vi "Read SPD (pps).vi"(8 "error in (no error)":errorcluster, 11 "Motor in":refnum<class "Motor.lvclass">) -> (0 "error out":errorcluster, 1 "min speed in pps":dbl, 2 "max speed in pps":dbl, 3 "Motor out":refnum<class "Motor.lvclass">)   [LabVIEW 2016, in "Hardware.lvlib" / "Motor.lvlib" / "Motor.lvclass"]
uses:
  <userlib>/Common Components/Hardware/Motor/Motor/Motor.lvclass
  <userlib>/Common Components/Hardware/Motor/Motor/Motor.lvclass/Motor.ctl
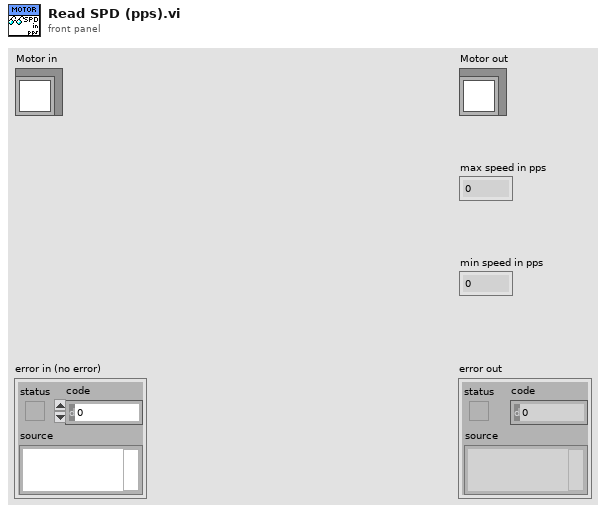
[diagram p1: front panel]
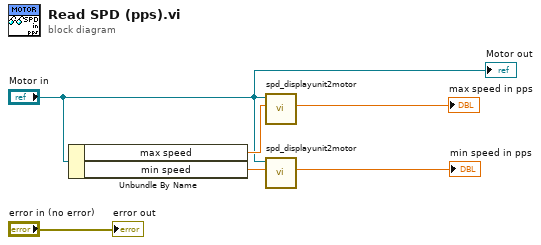
[diagram p0: block diagram]
diagram:
  n1 = Unbundle By Name("Motor in") -> ("max speed"=w5:dbl, "min speed"=w3:dbl)
  n2 = call <userlib>:"spd_displayunit2motor.vi"("speed in display unit/s"=w5, "Motor in"="Motor in") -> ("speed in pps"=→"max speed in pps":dbl)  [unwired: 7 in, 2 out]
  n3 = call <userlib>:"spd_displayunit2motor.vi"("speed in display unit/s"=w3, "Motor in"="Motor in") -> ("speed in pps"=→"min speed in pps":dbl)  [unwired: 7 in, 2 out]
  "error out" <- "error in (no error)"
  "Motor out" <- "Motor in"
